vi "FactorAnalysis.vi"(8 "error in":errorcluster) -> (0 "error out":errorcluster, 3 "out":refnum<class "FactorAnalysis.lvclass">)   [LabVIEW 2020]
doc: "Factor Analysis (FA).\n\n A simple linear generative model with Gaussian latent variables.\n\n The observations are assumed to be caused by a linear transformation of\n lower dimensional latent factors and added Gaussian noise.\n Without loss of generality the factors are distributed according to a\n Gaussian with zero mean and unit covariance. The noise is also zero mean\n and has an arbitrary diagonal covariance matrix.\n\n If we would restrict the model further, by assuming that the Gaussian\n noise is even isotropic (all diagonal entries are the same) we would obtain\n :class:`PPCA`.\n\n FactorAnalysis performs a maximum likelihood estimate of the so-called\n `loading` matrix, the transformation of the latent variables to the\n observed ones, using SVD based approach.\n\n Read more in the :ref:`User Guide <FA>`.\n\n .. versionadded:: 0.13\n\n Parameters\n ----------\n n_components : int, default=None\n Dimensionality of latent space, the number of components\n of ``X`` that are obtained after ``transform``.\n If None, n_components is set to the number of features.\n\n tol : float, defaul=1e-2\n Stopping tolerance for log-likelihood increase.\n\n copy : bool, default=True\n Whether to make a copy of X. If ``False``, the input X gets overwritten\n during fitting.\n\n max_iter : int, default=1000\n Maximum number of iterations.\n\n noise_variance_init : ndarray of shape (n_features,), default=None\n The initial guess of the noise variance for each feature.\n If None, it defaults to np.ones(n_features).\n\n svd_method : {'lapack', 'randomized'}, default='randomized'\n Which SVD method to use. If 'lapack' use standard SVD from\n scipy.linalg, if 'randomized' use fast ``randomized_svd`` function.\n Defaults to 'randomized'. For most applications 'randomized' will\n be sufficiently precise while providing significant speed gains.\n Accuracy can also be improved by setting higher values for\n `iterated_power`. If this is not sufficient, for maximum precision\n you should choose 'lapack'.\n\n iterated_power : int, default=3\n Number of iterations for the power method. 3 by default. Only used\n if ``svd_method`` equals 'randomized'.\n\n rotation : {'varimax', 'quartimax'}, default=None\n If not None, apply the indicated rotation. Currently, varimax and\n quartimax are implemented. See\n `\"The varimax criterion for analytic rotation in factor analysis\"\n <https://link.springer.com/article/10.1007%2FBF02289233>`_\n H. F. Kaiser, 1958.\n\n .. versionadded:: 0.24\n\n random_state : int or RandomState instance, default=0\n Only used when ``svd_method`` equals 'randomized'. Pass an int for\n reproducible results across multiple function calls.\n See :term:`Glossary <random_state>`.\n\n Attributes\n ----------\n components_ : ndarray of shape (n_components, n_features)\n Components with maximum variance.\n\n loglike_ : list of shape (n_iterations,)\n The log likelihood at each iteration.\n\n noise_variance_ : ndarray of shape (n_features,)\n The estimated noise variance for each feature.\n\n n_iter_ : int\n Number of iterations run.\n\n mean_ : ndarray of shape (n_features,)\n Per-feature empirical mean, estimated from the training set.\n\n \nAvailable methods:\nFit\nFit Transform\nTransform\nGet Attributes\nGet Params\nSet Params"
uses:
  FactorAnalysis.lvclass
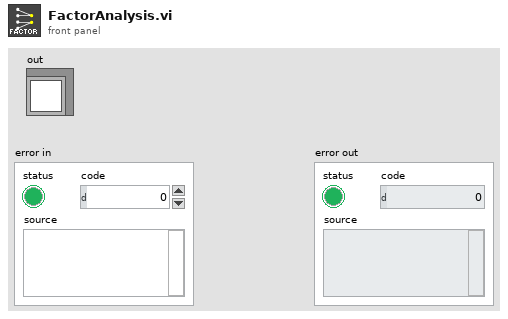
[diagram p1: front panel]
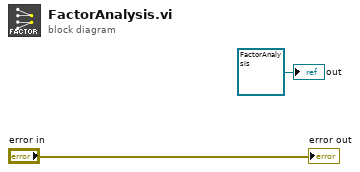
[diagram p0: block diagram]
diagram:
  "out" <- refnum<class "FactorAnalysis.lvclass"> refnum ("model")
  "error out" <- "error in"
